vi "Get API.vi"(8 "error in (no error)":errorcluster, 11 "TCPMessaging in":refnum<class "TCPMessaging.lvclass">) -> (0 "error out":errorcluster, 2 "TCP Messaging API":refnum<class "TCPMessageAPI.lvclass">, 3 "TCPMessaging out":refnum<class "TCPMessaging.lvclass">)   [LabVIEW 2020, in "Vecto.lvlib" / "TCPMessaging.lvclass"]
uses:
  TCPMessaging.lvclass
  TCPMessaging.lvclass/TCPMessaging.ctl
  TCPMessageService/TCPMessageAPI.lvclass
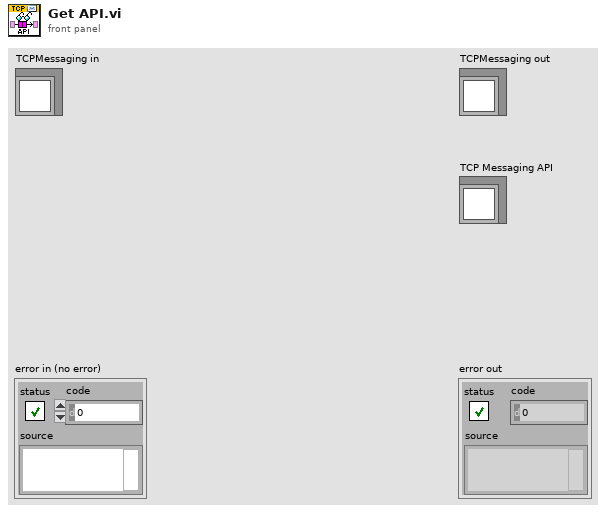
[diagram p1: front panel]
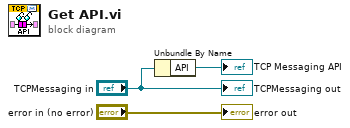
[diagram p0: block diagram]
diagram:
  n1 = Unbundle By Name("TCPMessaging in") -> ("API"=→"TCP Messaging API":refnum<class "TCPMessageAPI.lvclass">)
  "error out" <- "error in (no error)"
  "TCPMessaging out" <- "TCPMessaging in"
